vi "EMV Filter Non-High Temperatres F61.vi"(6 "T6 Temperature":dbl, 8 "error in (no error)":errorcluster, 9 "User Setpoint (0x4024) in":u16, 10 "Output in":T1) -> (0 "error out":errorcluster, 2 "Output out":T1)   [LabVIEW 2016]
uses:
  type defs/EMV Flow Stop Detection.ctl
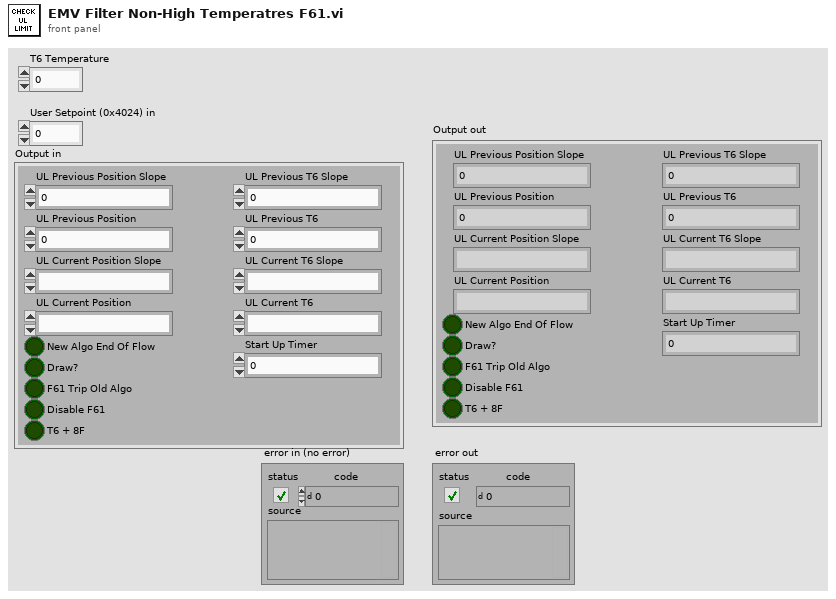
[diagram p1: front panel]
types:
  T1 = typedef "EMV Flow Stop Detection.ctl" = cluster{"UL Previous Position Slope":dbl, "UL Previous T6 Slope":dbl, "UL Previous Position":dbl, "UL Previous T6":dbl, "UL Current Position":dbl, "UL Current Position Slope":dbl, "UL Current T6":dbl, "UL Current T6 Slope":dbl, "New Algo End Of Flow":bool, "Start Up Timer":dbl, "Draw?":bool, "Disable F61":bool, "F61 Trip Old Algo":bool, "T6 + 8F":bool}
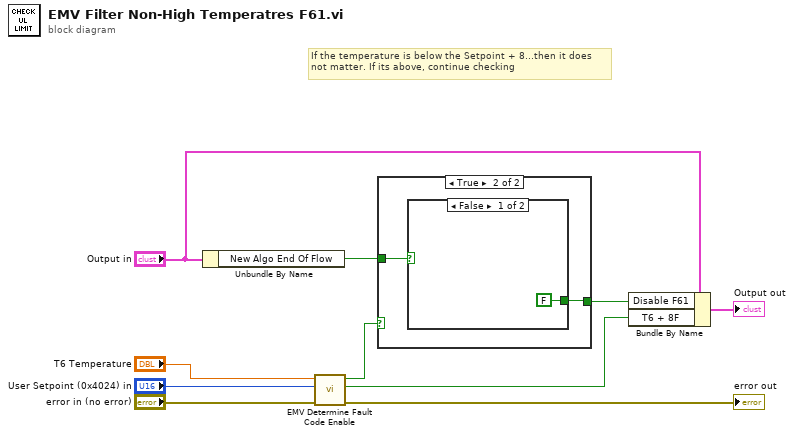
[diagram p0: block diagram]
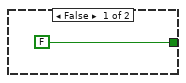
[diagram p2: hidden frame]
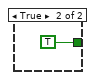
[diagram p3: hidden frame]
diagram:
  # "If the temperature is below the Setpoint + 8...then it does\nnot matter. If its above, continue checking"
  n1 = Unbundle By Name("Output in") -> ("New Algo End Of Flow"=w6:bool)
  n2 = call "EMV Determine Fault Code Enable.vi"("error in (no error)"="error in (no error)", "User Setpoint (0x4024) in"="User Setpoint (0x4024) in", "T6 Temperature"="T6 Temperature") -> ("error out"=→"error out":errorcluster, "> T6+8?"=w4:bool, "Disable F61?"=w7:bool)  [unwired: 6 in]
  n3 = case shown="True" w7 {
    tunnel: w6 -> [_ w13]
    tunnel: [FALSE ("End Of Flow") w12] -> w5
    frame False {
    }
    frame True {
      n4 = case shown="False" w13 {
        tunnel: [FALSE TRUE] -> w12
        frame False {
        }
        frame True {
        }
      }
    }
  }
  n5 = Bundle By Name(cluster="Output in", "Disable F61"=w5, "T6 + 8F"=w4) -> (→"Output out":T1)
